vi "Stage 2.1 myDAQ - Collecting A larger sample size.vi"() -> ()   [LabVIEW 2020]
panel:
  out "New Data":waveform(dbl)(graph)
  in  "Samples s":i32=5
  out "error out":errorcluster
  out "Raw":waveform(dbl)(graph)
  in  "Stop":bool
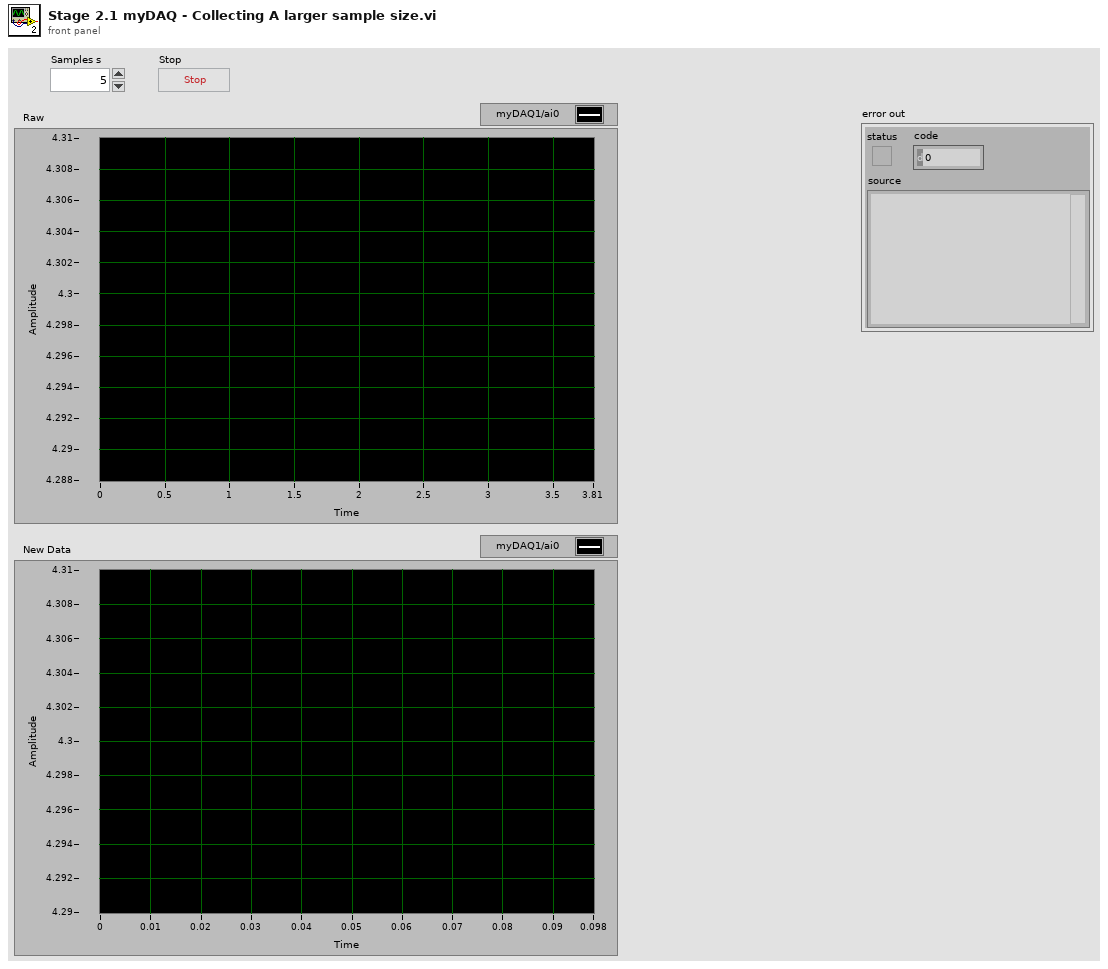
[diagram p1: front panel]
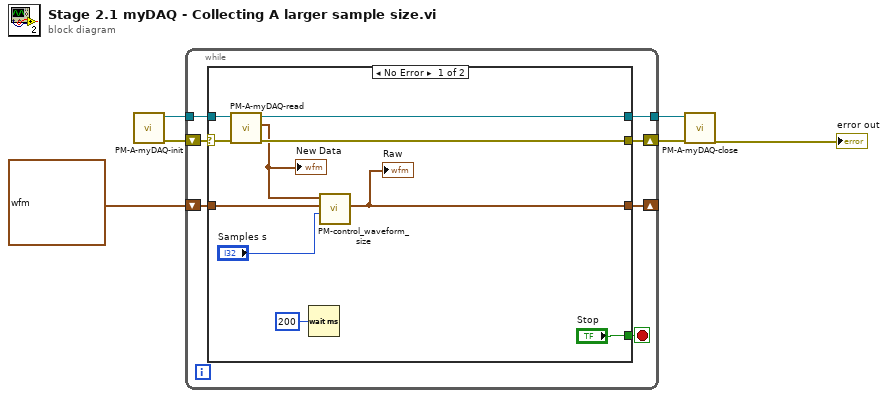
[diagram p0: block diagram]
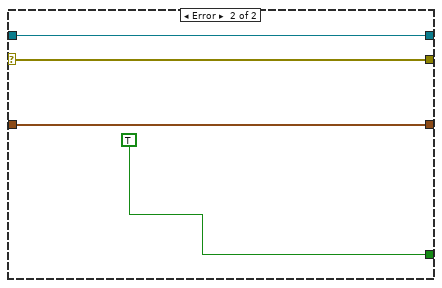
[diagram p2: hidden frame]
diagram:
  n1 = call "PM-A-myDAQ-init.vi"() -> ("error out"=w5:errorcluster, "Refnum out"=w4:refnum<k21>)  [unwired: 10 in]
  n2 = while {
    tunnel: w4 -> [w13]
    tunnel: [w11] -> w3
    shift-right: [w10] -> w2
    shift-left: w5 -> [w12]
    shift-right: [w7] -> _
    shift-left: waveform(dbl) {"t0"=timestamp(0 s since 1904-01-01), "dt"=0.0, "Y"=[]} ("data") -> [w8]
    stop <- w9 stop-if-true
    n3 = case shown="No Error" w12 {
      selector: w12 -> [w22 w26]
      tunnel: w13 -> [w23 w25]
      tunnel: [w20 w25] -> w11
      tunnel: [w19 w26] -> w10
      tunnel: ["Stop" TRUE ("Stop")] -> w9
      tunnel: w8 -> [w16 w24]
      tunnel: [w15 w24] -> w7
      frame No Error {
        n4 = call "PM-A-myDAQ-read.vi"("error in (no error)"=w22, "Refnum in"=w23) -> ("error out"=w19:errorcluster, "data"=w14:waveform(dbl), "Refnum out"=w20:refnum<k21>)  [unwired: 7 in]
        "New Data" <- w14
        n5 = Wait (ms)(milliseconds to wait=u32 200) -> ()  [unwired: 1 out]
        n6 = call "PM-control_waveform_size.vi"("Samples s"="Samples s", "old waveform"=w16, "New waveform"=w14) -> ("waveform"=w15:waveform(dbl))  [unwired: 8 in]
        "Raw" <- w15
      }
      frame Error {
      }
    }
  }
  n7 = call "PM-A-myDAQ-close.vi"("error in (no error)"=w2, "Refnum in"=w3) -> ("error out"=→"error out":errorcluster)  [unwired: 9 in]
